vi "Host - Download.vi"(8 "Error In (no error)":errorcluster, 9 "bitfile path in":path, 11 "Slave Ref in":refnum<k21>) -> (0 "error out":errorcluster, 1 "bitfile path out":path, 3 "Slave Ref out":refnum<k21>)   [LabVIEW 2019, in "SEECD System Explorer.lvlib"]
uses:
  SEECD System Explorer.lvlib
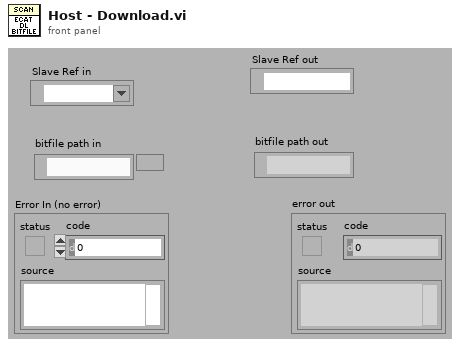
[diagram p1: front panel]
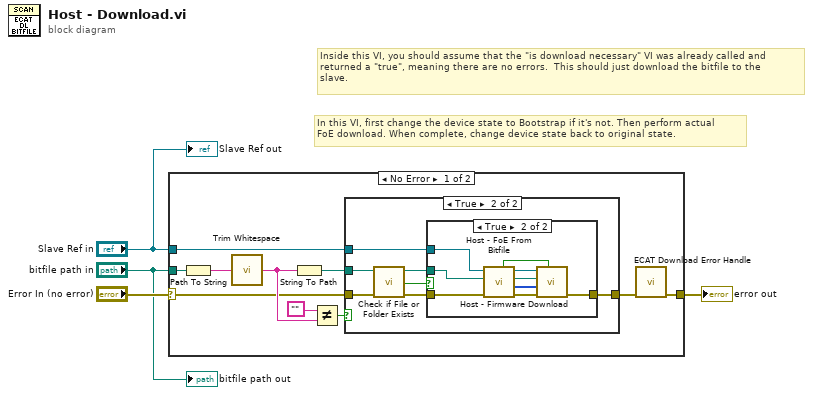
[diagram p0: block diagram]
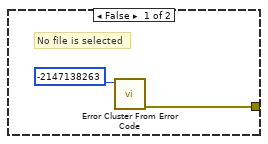
[diagram p2: hidden frame]
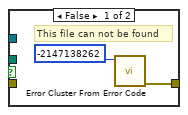
[diagram p3: hidden frame]
diagram:
  # "In this VI, first change the device state to Bootstrap if it's not. Then perform actual\nFoE download. When complete, change device state back to original state."
  # "Inside this VI, you should assume that the \"is download necessary\" VI was already called and\nreturned a \"true\", meaning there are no errors.  This should just download the bitfile to the\nslave."
  n1 = case shown="No Error" "Error In (no error)" {
    selector: "Error In (no error)" -> [w6 w35]
    tunnel: [w14 w35] -> w4
    tunnel: "bitfile path in" -> [w8 _]
    tunnel: "Slave Ref in" -> [w7 _]
    frame No Error {
      n2 = Path To String(path=w8) -> (string=w11:string)
      n3 = call <vilib>:"Trim Whitespace.vi"("string"=w11) -> ("trimmed string"=w13:string)  [unwired: 1 in]
      n4 = String To Path(string=w13) -> (path=w9:path)
      n5 = Not Equal?(x="", y=w13) -> (x != y?=w10:bool)
      n6 = case shown="True" w10 {
        tunnel: w7 -> [_ w23]
        tunnel: w9 -> [_ w22]
        tunnel: [w15 w18] -> w5
        tunnel: w6 -> [_ w17]
        frame False {
          # "No file is selected"
          n7 = call <vilib>:"Error Cluster From Error Code.vi"("error code (0)"=-2147138263) -> ("error out"=w15:errorcluster)  [unwired: 8 in]
        }
        frame True {
          n8 = call <vilib>:"Check if File or Folder Exists.vi"("error in (no error)"=w17, "path"=w22) -> ("error out"=w19:errorcluster, "file or folder exists?"=w21:bool, "dup path"=w20:path)  [unwired: 7 out]
          n9 = case shown="True" w21 {
            tunnel: w23 -> [_ w30]
            tunnel: w20 -> [_ w31]
            tunnel: w19 -> [_ w32]
            tunnel: [w24 w34] -> w18
            frame False {
              # "This file can not be found"
              n10 = call <vilib>:"Error Cluster From Error Code.vi"("error code (0)"=-2147138262) -> ("error out"=w24:errorcluster)  [unwired: 8 in]
            }
            frame True {
              n11 = call "Host - FoE From Bitfile.vi"("error in (no error)"=w32, "Firmware filename"=w31, "Slave Ref in"=w30) -> ("error out"=w33:errorcluster, "File Byte Array"=w28:u8[], "Firmware filename out"=w27:path, "Slave Ref out"=w29:refnum<k21>, "Need Reset"=w26:bool)  [unwired: 4 in]
              n12 = call "Host - Firmware Download.vi"("Need Reset"=w26, "error in (no error)"=w33, "File Byte Array"=w28, "Firmware filename"=w27, "Slave Ref in"=w29) -> ("error out"=w34:errorcluster)  [unwired: 6 in]
            }
          }
        }
      }
      n13 = call "ECAT Download Error Handle.vi"("error in"=w5) -> ("error out"=w14:errorcluster)  [unwired: 10 in]
    }
    frame Error {
    }
  }
  "error out" <- w4
  "bitfile path out" <- "bitfile path in"
  "Slave Ref out" <- "Slave Ref in"
